vi "3.90.3-Return FPGA Ref.vi"(1 "error in":errorcluster, 2 "Failed to Obtain Ref":bool, 3 "element":T1, 4 "FPGA Ref":refnum<queue>) -> (0 "error out":errorcluster)   [LabVIEW 2010]
doc: "Run this VI to safely return the reference to the FPGA you borrowed with the 3.90.2 vi"
uses:
  4-High Neurons/4.1-FPGA VI Typedef.ctl
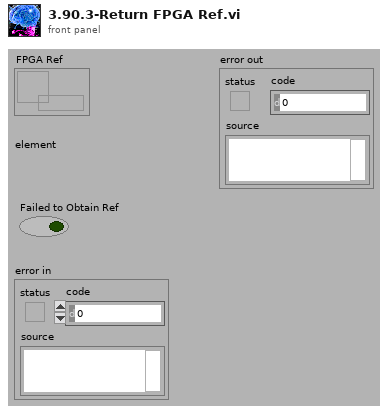
[diagram p1: front panel]
types:
  T1 = typedef "4.1-FPGA VI Typedef.ctl" = refnum<k20>
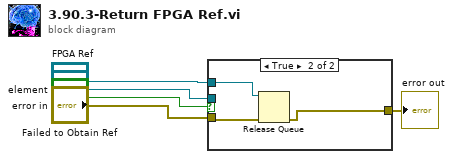
[diagram p0: block diagram]
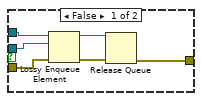
[diagram p2: hidden frame]
diagram:
  n1 = case shown="True" "Failed to Obtain Ref" {
    tunnel: "FPGA Ref" -> [w11 w14]
    tunnel: "element" -> [w10 _]
    tunnel: "error in" -> [w9 w13]
    tunnel: [w6 w12] -> w5
    frame False {
      n2 = Lossy Enqueue Element(queue=w11, element=w10, error in (no error)=w9) -> (queue out=w7:refnum<queue>, error out=w8:errorcluster)  [unwired: 2 out]
      n3 = Release Queue(queue=w7, error in (no error)=w8) -> (error out=w6:errorcluster)  [unwired: 1 in, 2 out]
    }
    frame True {
      n4 = Release Queue(queue=w14, error in (no error)=w13) -> (error out=w12:errorcluster)  [unwired: 1 in, 2 out]
    }
  }
  "error out" <- w5
